vi "ReadWindowsProperties.vi"(8 "ErrorIn":errorcluster, 11 "ReferenceIn":refnum<class "MasterGUI.lvclass">) -> (0 "ErrorOut":errorcluster, 2 "WindowsProperties":T1={"WindowsTitle"="", "Centered"=TRUE, "Minimizable"=FALSE, "State"=enum."Standard", "Position"={"X"=200, "Y"=200}, "Size"={"X"=800, "Y"=600}}, 3 "ReferenceIn":refnum<class "MasterGUI.lvclass">)   [LabVIEW 2021, in "MasterGUI.lvclass"]
uses:
  MasterGUI.lvclass
  MasterGUI.lvclass/MasterGUI.ctl
  WindowsProperties.ctl
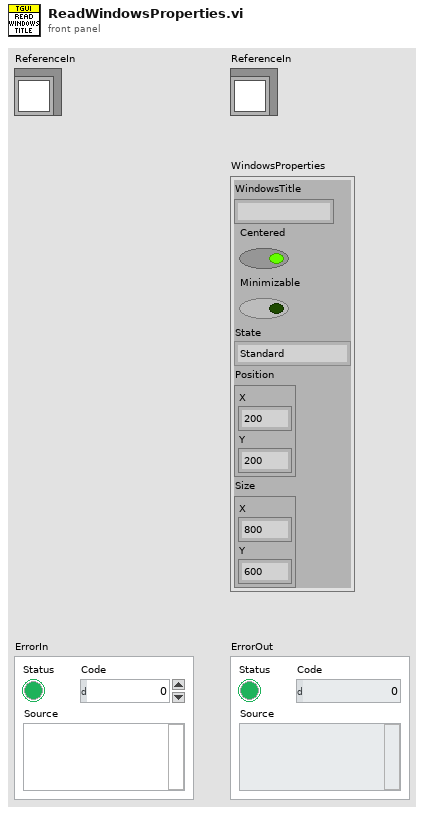
[diagram p1: front panel]
types:
  T1 = typedef "MasterGUI.lvclass/WindowsProperties.ctl" = cluster{"WindowsTitle":string, "Centered":bool, "Minimizable":bool, "State":enum32{"Invalid", "Standard", "Closed", "Hidden", "Minimized", "Maximized"}, "Position":cluster{"X":i32, "Y":i32}, "Size":cluster{"X":i32, "Y":i32}}
  T2 = typedef "MasterGUI.lvclass/ObjectAttributes.ctl" = cluster{"Interfaces":cluster{"Dummy":refnum<class>}, "Locals":cluster{"MainGUIActive":refnum<queue>, "MainPanel":refnum<vi>, "LayoutPanel":cluster{"PanelVIRef":refnum<vi>, "Labels":string[], "SubPanels":refnum<vi>[]}, "MenuTree":T3[], "Menu":refnum<k9>}, "Persistent":cluster{"StaticDocking":cluster{"ObjectLabel":string, "SubPanelLabel":string}[], "WindowsProperties":T1, "AdditionalMenuItems":T3[], "TraceObjectName":string}}
  T3 = typedef "MasterGUI.lvclass/MenuItem.ctl" = cluster{"Parent":string, "Items":string[], "ShortCuts":cluster{"IncludeShiftKey":bool, "IncludeCtrlKey":bool, "ShortcutKey":string}[]}
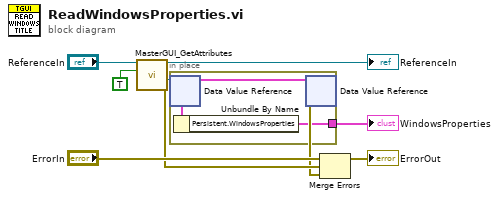
[diagram p0: block diagram]
diagram:
  n1 = call "MasterGUI_GetAttributes.vi"("OnlyGetDvrReference(False)"=TRUE, "ReferenceIn"="ReferenceIn") -> ("ErrorOut"=w8:errorcluster, "DataRef"=w2:refnum<data-value>, "ReferenceOut"=→"ReferenceIn":refnum<class "MasterGUI.lvclass">)  [unwired: 6 in, 1 out]
  n2 = in-place {
    in-place-border: [w11] -> w1
    n3 = in-place-dvr #1(w2) -> (w10:T2)  [unwired: 1 out]
    n4 = Unbundle By Name(w10) -> ("Persistent.WindowsProperties"=w11:T1)
    n5 = in-place-dvr #1(w10) -> (w6:errorcluster)  [unwired: 1 out]
  }
  "WindowsProperties" <- w1
  n6 = Merge Errors("ErrorIn", w8, w6) -> (→"ErrorOut":errorcluster)
